vi "propagation.vi"() -> ()   [LabVIEW 2020]
uses:
  <vilib>/Utility/file.llb/Read Delimited Spreadsheet (DBL).vi
  <vilib>/Analysis/1siggen.llb/Ramp Pattern by Delta.vi
  <vilib>/Analysis/NI_AALBase.lvlib
  <vilib>/gmath/NI_Gmath.lvlib
panel:
  out "Array":dbl[](array[numeric])
  out "보간후":cluster{"all rows":dbl[], "all rows":dbl[]}(graph)
  out "sqrt(x)":dbl
  out "보간전":cluster{"all rows":dbl[], "all rows":dbl[]}(graph)
  out "samples":i32
  in  "Numeric":i32
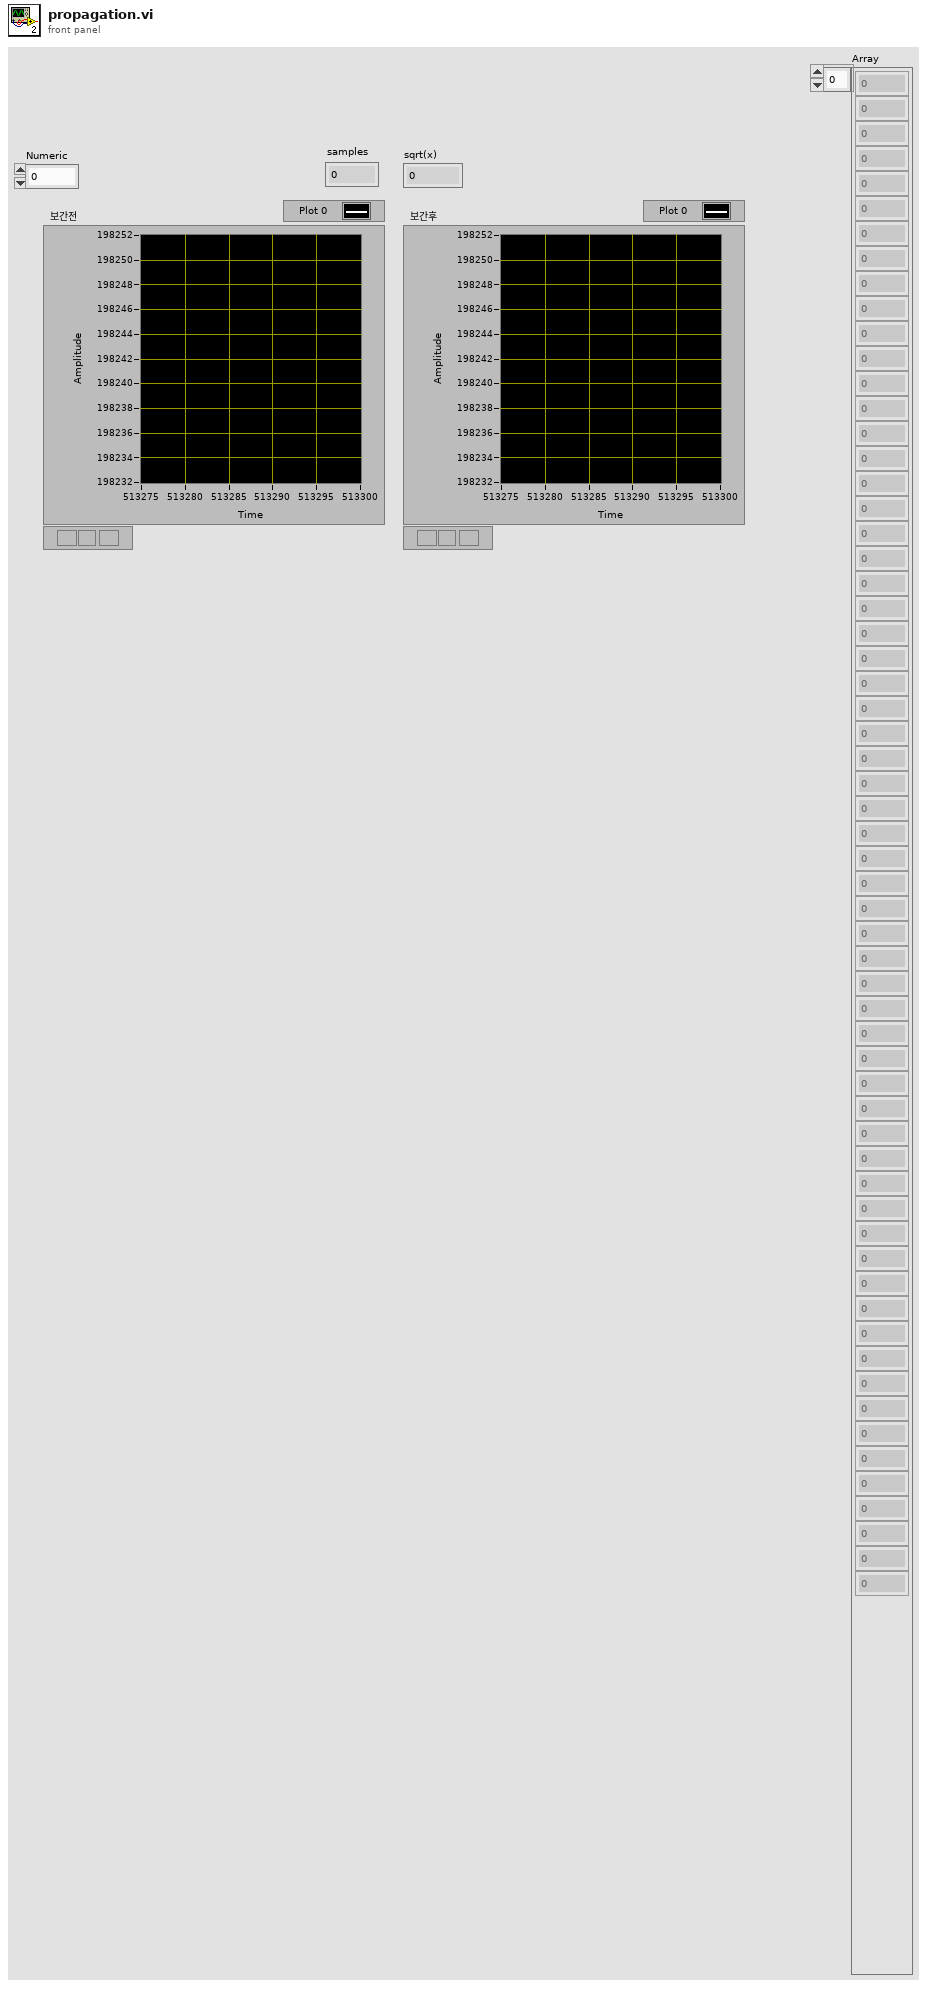
[diagram p1: front panel]
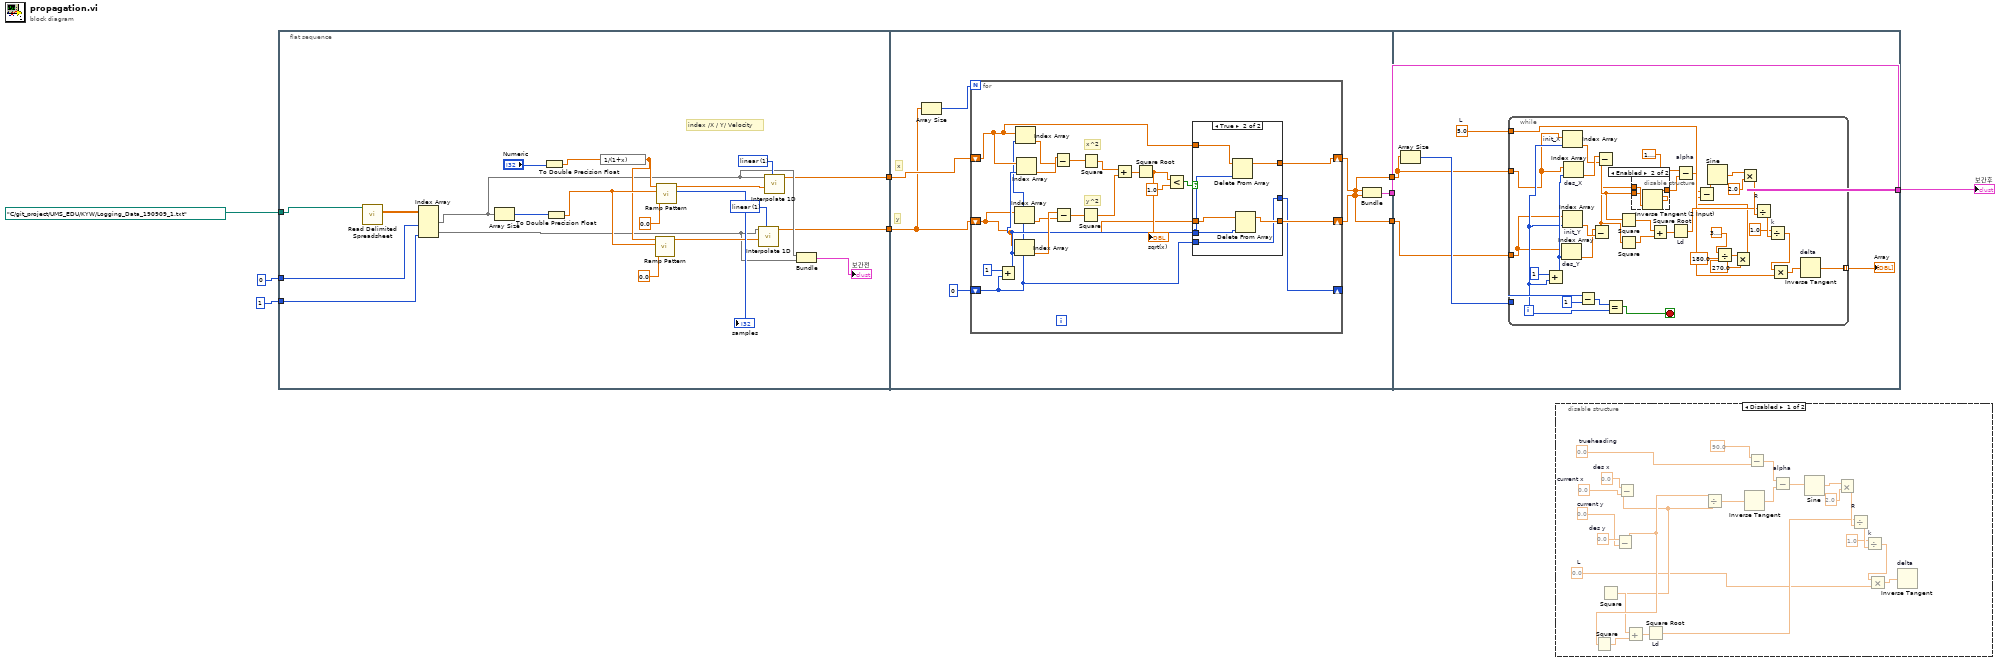
[diagram p0: block diagram]
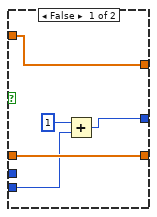
[diagram p3: hidden frame]
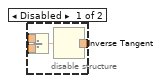
[diagram p4: hidden frame]
diagram:
  n1 = flat-sequence {
    tunnel: path "C:/git_project/UMS_EDU/KYW/Logging_Data_190909_1.txt" ("name or relative path") -> [w12]
    tunnel: [w14] -> w8
    tunnel: [w13] -> w7
    tunnel: 1 ("index (col)") -> [w11]
    tunnel: 0 ("disabled index (col)") -> [w10]
    tunnel: w8 -> [w35]
    tunnel: w7 -> [w34]
    tunnel: [w37] -> w3
    tunnel: [w32] -> w2
    tunnel: [w31] -> w1
    tunnel: [w74] -> w6
    tunnel: w3 -> [w74]
    tunnel: w2 -> [w72]
    tunnel: w1 -> [w71]
    frame #0 {
      w29 = 1 items=["nearest", "linear", "spline", "cubic Hermite", "Lagrange"] ("method")
      w28 = 1 items=["nearest", "linear", "spline", "cubic Hermite", "Lagrange"] ("method")
      # "index /X / Y/ Velocity"
      n2 = call-poly <vilib>:"Read Delimited Spreadsheet.vi"("file path (dialog if empty)"=w12) -> ("all rows"=w30:dbl[][])  [unwired: 9 in, 5 out]
      n3 = Index Array(array=w30, index (col) #1=w10, index (col) #2=w11) -> (element #1=w15:dbl[], element #2=w16:dbl[])  [unwired: 2 in]
      n4 = Array Size(array=w15) -> (size(s)=w27:i32)
      n5 = To Double Precision Float(number="Numeric") -> (double precision float=w21:dbl)
      n6 = To Double Precision Float(number=w27) -> (double precision float=w26:dbl)
      n7 = expression code="1/(1+x)"(w21) -> (w23:dbl)
      n8 = call-poly <vilib>:"Ramp Pattern.vi"("start"=0.0, "end"=w26, "delta"=w23) -> ("Ramp Pattern"=w18:dbl[])  [unwired: 6 in, 2 out]
      n9 = call-poly <vilib>:"Ramp Pattern.vi"("start"=0.0, "end"=w26, "delta"=w23) -> ("samples"=→"samples":i32, "Ramp Pattern"=w19:dbl[])  [unwired: 6 in, 1 out]
      n10 = call <vilib>:"Interpolate 1D.vi"("method"=w28, "xi"=w18, "Y"=w16) -> ("yi"=w13:dbl[])  [unwired: 6 in, 2 out]
      n11 = call <vilib>:"Interpolate 1D.vi"("method"=w29, "xi"=w19, "Y"=w15) -> ("yi"=w14:dbl[])  [unwired: 6 in, 2 out]
      n12 = Bundle("all rows"=w15, "all rows"=w16) -> (→"보간전":cluster{"all rows":dbl[], "all rows":dbl[]})  [unwired: 1 in]
    }
    frame #1 {
      # "y"
      # "x"
      n13 = Array Size(array=w34) -> (size(s)=w33:i32)
      n14 = for {
        N: w33 -> [_]
        shift-right: [w45] -> w31
        shift-left: w34 -> [w38]
        shift-right: [w46] -> w32
        shift-left: w35 -> [w40]
        shift-right: [w44] -> _
        shift-left: 0 ("x") -> [w39]
        # "y^2"
        # "x^2"
        n15 = Add(x=1, y=w39) -> (x+y=w47:i32)
        n16 = Index Array(array=w38, index=w47) -> (element=w55:dbl)
        n17 = Index Array(array=w38, index=w39) -> (element=w49:dbl)
        n18 = Index Array(array=w40, index=w39) -> (element=w48:dbl)
        n19 = Index Array(array=w40, index=w47) -> (element=w56:dbl)
        n20 = Subtract(x=w56, y=w48) -> (x-y=w53:dbl)
        n21 = Subtract(x=w55, y=w49) -> (x-y=w54:dbl)
        n22 = Square(x=w54) -> (x^2=w52:dbl)
        n23 = Square(x=w53) -> (x^2=w51:dbl)
        n24 = Add(x=w51, y=w52) -> (x+y=w50:dbl)
        n25 = Square Root(x=w50) -> (sqrt(x)=w43:dbl)
        "sqrt(x)" <- w43
        n26 = Less?(x=w43, y=1.0) -> (x < y?=w41:bool)
        n27 = case shown="True" w41 {
          tunnel: w40 -> [w59 w68]
          tunnel: w47 -> [_ w65]
          tunnel: [w59 w67] -> w46
          tunnel: [w62 w66] -> w45
          tunnel: w38 -> [w62 w64]
          tunnel: [w60 w63] -> w44
          tunnel: w39 -> [w58 w63]
          frame False {
            n28 = Add(x=1, y=w58) -> (x+y=w60:i32)
          }
          frame True {
            n29 = Delete From Array(array=w68, index=w65) -> (array with subset deleted=w67:dbl[])  [unwired: 1 in, 1 out]
            n30 = Delete From Array(array=w64, index=w65) -> (array with subset deleted=w66:dbl[])  [unwired: 1 in, 1 out]
          }
        }
      }
      n31 = Bundle("yi"=w32, "yi"=w31) -> (w37:cluster{"yi":dbl[], "yi":dbl[]})  [unwired: 1 in]
    }
    frame #2 {
      w70 = 5.0  # L
      n32 = Array Size(array=w72) -> (size(s)=w73:i32)
      n33 = while {
        tunnel: w73 -> [w110]
        tunnel: w72 -> [w104]
        tunnel: w71 -> [w103]
        tunnel: w70 -> [w85]
        tunnel: [w83] -> w69 mode=indexing
        i -> [w105]
        stop <- w111 stop-if-true
        n34 = Add(x=1, y=w105) -> (x+y=w106:i32)
        n35 = Index Array "des_Y"(array=w103, index=w106) -> (element=w99:dbl)
        n36 = Index Array "init_Y"(array=w103, index=w105) -> (element=w100:dbl)
        n37 = Index Array "init_X"(array=w104, index=w105) -> (element=w101:dbl)
        n38 = Index Array "des_X"(array=w104, index=w106) -> (element=w102:dbl)
        n39 = Subtract(x=w110, y=1) -> (x-y=w108:i32)
        n40 = Subtract(x=w99, y=w100) -> (x-y=w96:dbl)
        n41 = Subtract(x=w102, y=w101) -> (x-y=w97:dbl)
        n42 = Equal?(x=w108, y=w105) -> (x = y?=w111:bool)
        n43 = Square(x=w97) -> (x^2=w95:dbl)
        n44 = Square(x=w96) -> (x^2=w94:dbl)
        n45 = disable-structure shown="Enabled" {
          disable-tunnel: [w115 w116] -> w98
          disable-tunnel: w97 -> [w114 w117]
          disable-tunnel: w96 -> [w113 w118]
          frame Disabled {
            n46 = Divide(x=w113, y=w114) -> (x/y=w112:dbl)
            n47 = Inverse Tangent(1:w112) -> (0:w115:dbl)
          }
          frame Enabled {
            n48 = Inverse Tangent (2 Input)(1:w118, 2:w117) -> (0:w116:dbl)
          }
        }
        n49 = Add(x=w95, y=w94) -> (x+y=w93:dbl)
        n50 = Square Root "Ld"(x=w93) -> (sqrt(x)=w89:dbl)
        n51 = Subtract "alpha"(x=1.5707963267948966, y=w98) -> (x-y=w76:dbl)
        n52 = Divide(x=3.141592653589793, y=180.0) -> (x/y=w79:dbl)
        n53 = Multiply(x=w79, y=270.0) -> (x*y=w77:dbl)
        n54 = Subtract(x=w76, y=w77) -> (x-y=w75:dbl)
        n55 = Sine(x=w75) -> (sin(x)=w92:dbl)
        n56 = Multiply(x=w92, y=2.0) -> (x*y=w90:dbl)
        n57 = Divide "R"(x=w89, y=w90) -> (x/y=w88:dbl)
        n58 = Divide "k"(x=1.0, y=w88) -> (x/y=w86:dbl)
        n59 = Multiply(x=w86, y=w85) -> (x*y=w84:dbl)
        n60 = Inverse Tangent "delta"(1:w84) -> (0:w83:dbl)
      }
      "Array" <- w69
    }
  }
  n61 = disable-structure shown="Disabled" {
    frame Disabled {
      w119 = 0.0  # L
      w121 = 0.0  # trueheading
      w124 = 0.0  # current y
      w125 = 0.0  # des y
      w126 = 0.0  # current x
      w127 = 0.0  # des x
      n62 = Subtract(x=w125, y=w124) -> (x-y=w141:dbl)
      n63 = Square(x=w141) -> (x^2=w139:dbl)
      n64 = Subtract(x=w127, y=w126) -> (x-y=w123:dbl)
      n65 = Square(x=w123) -> (x^2=w140:dbl)
      n66 = Add(x=w140, y=w139) -> (x+y=w138:dbl)
      n67 = Square Root "Ld"(x=w138) -> (sqrt(x)=w133:dbl)
      n68 = Divide(x=w141, y=w123) -> (x/y=w128:dbl)
      n69 = Inverse Tangent(1:w128) -> (0:w142:dbl)
      n70 = Subtract(x=90.0, y=w121) -> (x-y=w120:dbl)
      n71 = Subtract "alpha"(x=w120, y=w142) -> (x-y=w137:dbl)
      n72 = Sine(x=w137) -> (sin(x)=w136:dbl)
      n73 = Multiply(x=w136, y=2.0) -> (x*y=w134:dbl)
      n74 = Divide "R"(x=w133, y=w134) -> (x/y=w132:dbl)
      n75 = Divide "k"(x=1.0, y=w132) -> (x/y=w130:dbl)
      n76 = Multiply(x=w130, y=w119) -> (x*y=w129:dbl)
      n77 = Inverse Tangent "delta"(1:w129) -> ()  [unwired: 1 out]
    }
    frame Enabled {
    }
  }
  "보간후" <- w6
